vi "Read Write Text File Test.vi"(8 "Error In":errorcluster) -> (0 "Error Out":errorcluster)   [LabVIEW 2023, in "Test.lvlib"]
doc: "The VI is a test file to test the functionality of read and write text files."
uses:
  Test.lvlib
  File Path Operations/Controls/FileOperation.ctl
  <vilib>/addons/_JKI Toolkits/Caraya/classes/Assert/Assert Equal Value_Variant.vi
  <vilib>/addons/_JKI Toolkits/Caraya/classes/Assert/Assert.lvclass
  <vilib>/addons/_JKI Toolkits/Caraya/classes/Test/Test.lvclass
  File Path Operations/File and Path Operations.lvlib
panel:
  # "READ WRITE TEXT FILE TEST"
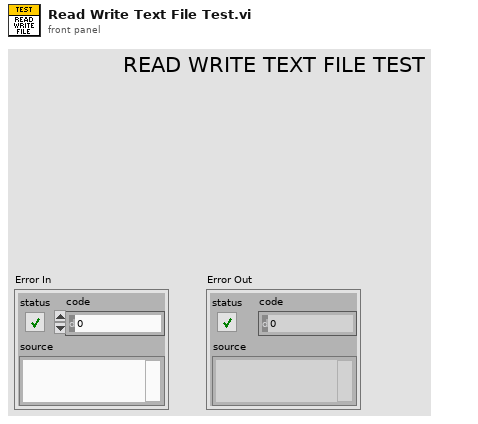
[diagram p1: front panel]
types:
  T1 = typedef "File and Path Operations.lvlib/FileOperation.ctl" = enum16{"Read", "Write"}
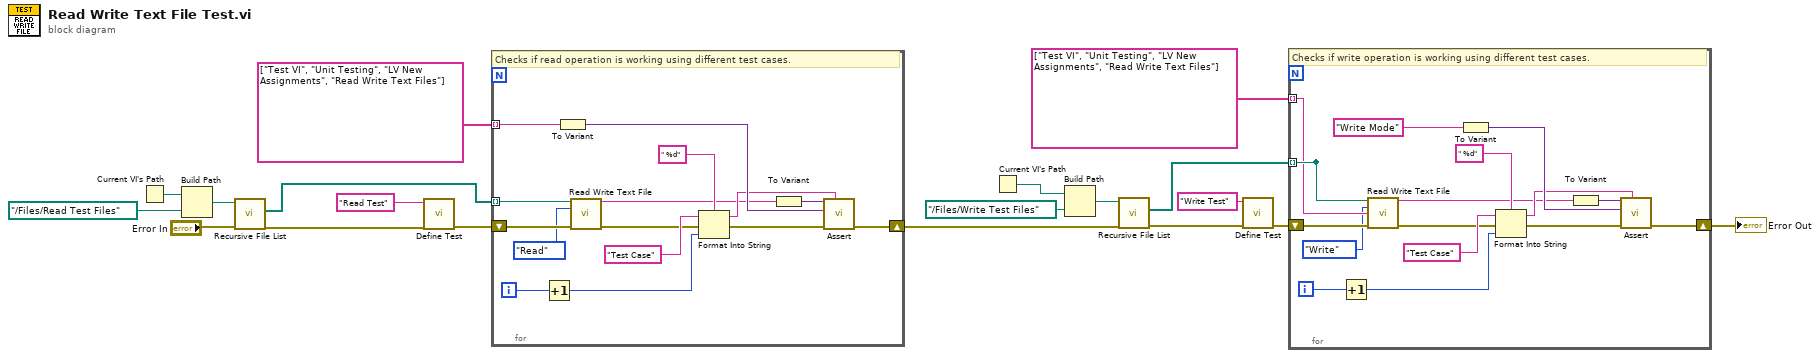
[diagram p0: block diagram]
diagram:
  n1 = Current VI's Path() -> (path=w1:path)
  n2 = Build Path(base path=w1, name or relative path=path "../Files/Read Test Files") -> (appended path=w15:path)
  n3 = call <vilib>:"Recursive File List.vi"("error in (no error)"="Error In", "Folder Path"=w15) -> ("error out"=w14:errorcluster, "All Files in Dir"=w13:path[])  [unwired: 5 in, 3 out]
  n4 = call <vilib>:"Define Test.vi"("error in (no error)"=w14, "Label (VI Title)"="Read Test") -> ("error out"=w17:errorcluster)  [unwired: 8 in, 1 out]
  n5 = for {
    tunnel: w13 -> [w21] mode=indexing
    shift-right: [w23] -> w9
    shift-left: w17 -> [w26]
    tunnel: string[] ["Test VI", "Unit Testing", "LV New Assignments", "Read Write Text Files"] ("Array") -> [w34] mode=indexing
    i -> [w29]
    # "Checks if read operation is working using different test cases."
    n6 = Increment(x=w29) -> (x+1=w24:i32)
    n7 = To Variant(anything=w34) -> (Variant=w33:variant)
    n8 = call "Read Write Text File.vi"("File Path"=w21, "File Operation"=FileOperation."Read", "Error In"=w26) -> ("Text Output"=w22:string, "Error Out"=w25:errorcluster)  [unwired: 11 in]
    n9 = Format Into String(format string=" %d", initial string="Test Case" ("Label"), error in=w25, w24) -> (resulting string=w27:string, error out=w31:errorcluster)
    n10 = To Variant(anything=w22) -> (Variant=w32:variant)
    n11 = call-poly <vilib>:"Assert.vi"("Label"=w27, "error in (no error)"=w31, "Y"=w33, "X"=w32) -> ("error out"=w23:errorcluster)  [unwired: 6 in, 1 out]
  }
  n12 = Current VI's Path() -> (path=w2:path)
  n13 = Build Path(base path=w2, name or relative path=path "../Files/Write Test Files") -> (appended path=w6:path)
  n14 = call <vilib>:"Recursive File List.vi"("error in (no error)"=w9, "Folder Path"=w6) -> ("error out"=w8:errorcluster, "All Files in Dir"=w7:path[])  [unwired: 5 in, 3 out]
  n15 = call <vilib>:"Define Test.vi"("error in (no error)"=w8, "Label (VI Title)"="Write Test") -> ("error out"=w11:errorcluster)  [unwired: 8 in, 1 out]
  n16 = for {
    tunnel: [w38] -> _ mode=indexing
    shift-right: [w40] -> w3
    shift-left: w11 -> [w43]
    tunnel: w7 -> [w38] mode=indexing
    tunnel: string[] ["Test VI", "Unit Testing", "LV New Assignments", "Read Write Text Files"] ("Array") -> [w37] mode=indexing
    i -> [w46]
    # "Checks if write operation is working using different test cases."
    n17 = Increment(x=w46) -> (x+1=w41:i32)
    n18 = call "Read Write Text File.vi"("File Path"=w38, "File Operation"=FileOperation."Write", "Text Input"=w37, "Error In"=w43) -> ("Text Output"=w39:string, "Error Out"=w42:errorcluster)  [unwired: 10 in]
    n19 = To Variant(anything="Write Mode" ("File/Folder Name")) -> (Variant=w50:variant)
    n20 = Format Into String(format string=" %d", initial string="Test Case" ("Label"), error in=w42, w41) -> (resulting string=w44:string, error out=w48:errorcluster)
    n21 = To Variant(anything=w39) -> (Variant=w49:variant)
    n22 = call-poly <vilib>:"Assert.vi"("Label"=w44, "error in (no error)"=w48, "Y"=w50, "X"=w49) -> ("error out"=w40:errorcluster)  [unwired: 6 in, 1 out]
  }
  "Error Out" <- w3
